vi "Write formatString.vi"(8 "error in (no error)":errorcluster, 10 "formatString":string, 11 "Tag in":refnum<class "Tag.lvclass">) -> (0 "error out":errorcluster, 3 "Tag out":refnum<class "Tag.lvclass">)   [LabVIEW 2020, in "Tag Engine Core.lvlib" / "Tag.lvclass"]
doc: "_SubVI_"
uses:
  Tag.lvclass
  Tag.lvclass/Tag.ctl
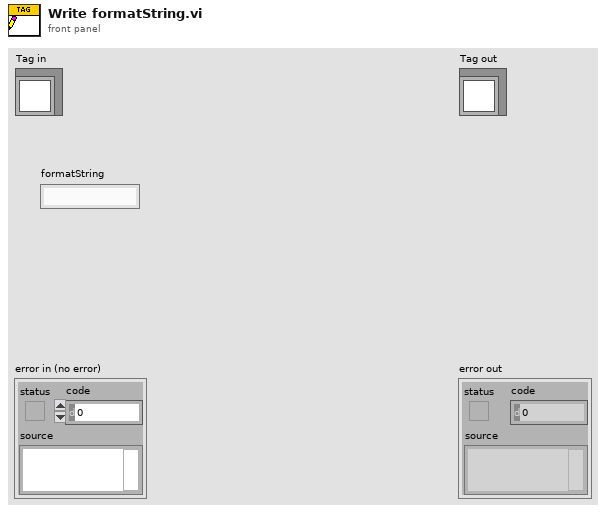
[diagram p1: front panel]
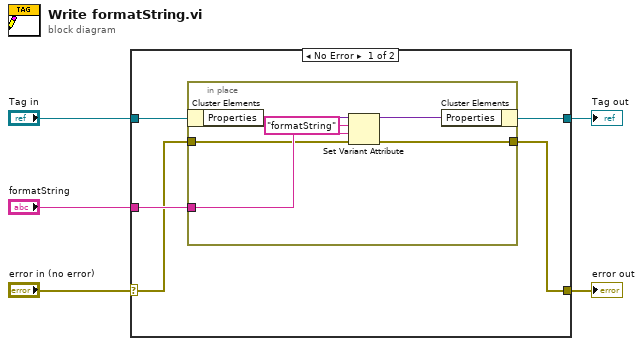
[diagram p0: block diagram]
diagram:
  n1 = case shown="No Error" "error in (no error)" {
    selector: "error in (no error)" -> [w7 w17]
    tunnel: [w6 w17] -> w4
    tunnel: [w9 w18] -> w2
    tunnel: "Tag in" -> [w10 w18]
    tunnel: "formatString" -> [w8 _]
    frame No Error {
      n2 = in-place {
        in-place-border: w8 -> [w13]
        in-place-border: w7 -> [w12]
        in-place-border: [w11] -> w6
        n3 = in-place-cluster #1(w10) -> ("Properties"=w16:variant)
        n4 = Set Variant Attribute(Variant=w16, name="formatString", value=w13, error in=w12) -> (Variant out=w14:variant, error out=w11:errorcluster)  [unwired: 1 out]
        n5 = in-place-cluster #1("Properties"=w14) -> (w9:refnum<class "Tag.lvclass">)
      }
    }
    frame Error {
    }
  }
  "error out" <- w4
  "Tag out" <- w2
